vi "LoadDriveValues.vi"(8 "error in":errorcluster) -> (0 "error out":errorcluster)   [LabVIEW 2015]
uses:
  Drive/Implementation/Advanced Drive VIs/PID Type Def.ctl
  <vilib>/Rock Robotics/Network Tables/NT Read Numeric Array.vi
  Drive/Implementation/RobotDriveGlobal.vi
panel:
  out "Speed PID":T1
  out "Distance PID":T1
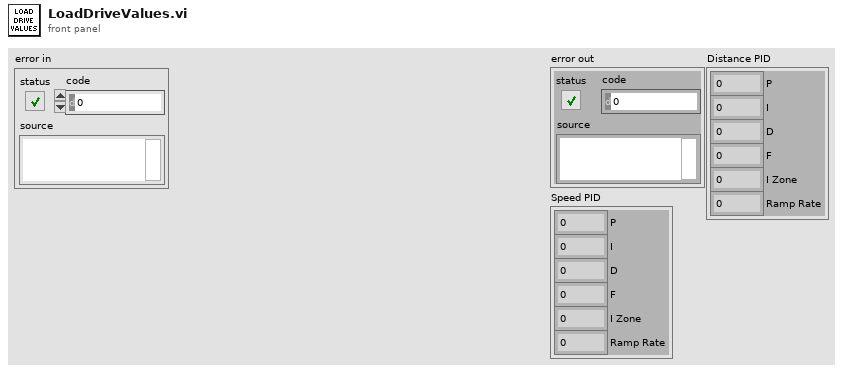
[diagram p1: front panel]
types:
  T1 = typedef "PID Type Def.ctl" = cluster{"P":dbl, "I":dbl, "D":dbl, "F":dbl, "I Zone":dbl, "Ramp Rate":dbl}
  T2 = typedef "RobotDrive Type Def.ctl" = cluster{"RobotDriveDevRef":cluster{"DevStatus":errorcluster, "Motors[]":T3[], "Square Inputs":bool, "Max Output":dbl}, "Control Mode":T9, "Motor Settings":T10, "Default Control Mode":T9, "Speed Mag":dbl}
  T3 = typedef "WPI_MotorControlDeviceRef.ctl" = cluster{"DeviceStatus":errorcluster, "Type":T4, "PWM":cluster{"PWM Channel":T5, "DeadBand":T6}, "CAN":cluster{"Device Number":u8, "Control Mode":T7, "Semaphore":T8, "Max Vout":dbl, "TalonSRX Control Mode":T9}, "Invert":bool}
  T4 = typedef "WPI_MotorControlType.ctl" = enum16{"PWM", "CAN", "CANTalonSRX"}
  T5 = typedef "FPGA_DIOPWMChannel.ctl" = enum8{"PWM 0", "PWM 1", "PWM 2", "PWM 3", "PWM 4", "PWM 5", "PWM 6", "PWM 7", "PWM 8", "PWM 9", "PWM MXP 0", "PWM MXP 1", "PWM MXP 2", "PWM MXP 3", "PWM MXP 4", "PWM MXP 5", "PWM MXP 6", "PWM MXP 7", "PWM MXP 8", "PWM MXP 9", "Invalid"}
  T6 = typedef "WPI_PWMDeadband.ctl" = cluster{"Name":string, "maxPositivePwm":i32, "minPositivePwm":i32, "centerPwm":i32, "maxNegativePwm":i32, "minNegativePwm":i32, "angularRange":u16}
  T7 = typedef "WPI_CANJaguar_ControlMode.ctl" = enum8{"Percent VBus", "Current", "Speed", "Position", "Voltage"}
  T8 = typedef "Semaphore RefNum" = refnum<k1>
  T9 = typedef "WPI_CANTalonSRX_APIControlMode.ctl" = enum8{"Percent VBus", "Speed", "Position", "Slave", "Unchanged / Invalid", "Voltage Compensation", "Current", "Motion Profile"}
  T10 = typedef "Drive Motor Settings.ctl" = cluster{"Wheel Radius":dbl, "Encoder Ticks Per Rev":dbl, "Gear Ratio":dbl, "ClimbRev":dbl}
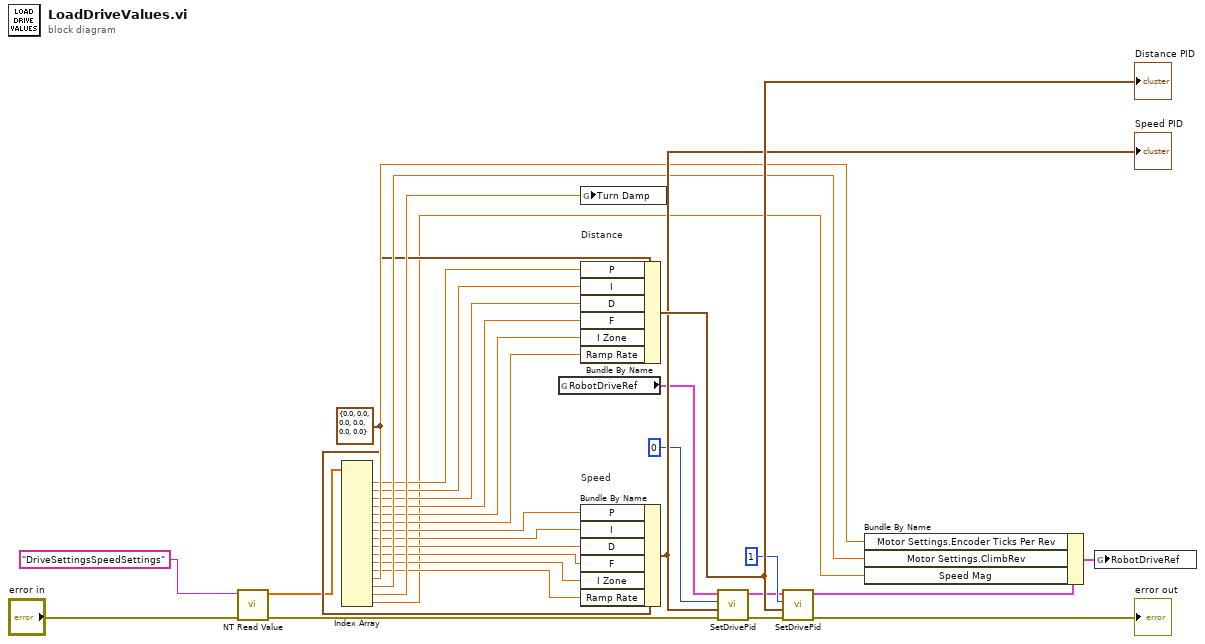
[diagram p0: block diagram]
diagram:
  w14 = T1 {"P"=0.0, "I"=0.0, "D"=0.0, "F"=0.0, "I Zone"=0.0, "Ramp Rate"=0.0} ("PID")
  n1 = call-poly <vilib>:"NT Read Value.vi"("error in"="error in", "Name"="DriveSettingsSpeedSettings") -> ("error out"=w3:errorcluster, "Numeric Array"=w7:dbl[])  [unwired: 8 in]
  n2 = Index Array(array=w7) -> (element #1=w8:dbl, element #2=w9:dbl, element #3=w10:dbl, element #4=w11:dbl, element #5=w12:dbl, element #6=w13:dbl, element #7=w15:dbl, element #8=w16:dbl, element #9=w17:dbl, element #10=w18:dbl, element #11=w19:dbl, element #12=w20:dbl, element #13=w28:dbl, element #14=w27:dbl, element #15=w31:dbl, element #16=w1:dbl)  [unwired: 16 in]
  n3 = global read "RobotDriveGlobal.vi" "RobotDriveRef"() -> (w21:T2)
  n4 = global write "RobotDriveGlobal.vi" "Turn Damp"(w31) -> ()
  n5 = Bundle By Name "Distance"(cluster=w14, "P"=w8, "I"=w9, "D"=w10, "F"=w11, "I Zone"=w12, "Ramp Rate"=w13) -> (w30:T1)
  "Distance PID" <- w30
  n6 = Bundle By Name "Speed"(cluster=w14, "P"=w15, "I"=w16, "D"=w17, "F"=w18, "I Zone"=w19, "Ramp Rate"=w20) -> (w29:T1)
  "Speed PID" <- w29
  n7 = call "SetDrivePid.vi"("error in (no error)"=w3, "PID"=w29, "Profile Slot"=u8 0, "RobotDriveRef In"=w21) -> ("error out"=w4:errorcluster, "RobotDriveRef Out"=w23:T2)  [unwired: 6 in]
  n8 = call "SetDrivePid.vi"("error in (no error)"=w4, "PID"=w30, "Profile Slot"=u8 1, "RobotDriveRef In"=w23) -> ("error out"=→"error out":errorcluster, "RobotDriveRef Out"=w25:T2)  [unwired: 6 in]
  n9 = Bundle By Name(cluster=w25, "Motor Settings.Encoder Ticks Per Rev"=w28, "Motor Settings.ClimbRev"=w27, "Speed Mag"=w1) -> (w26:T2)
  n10 = global write "RobotDriveGlobal.vi" "RobotDriveRef"(w26) -> ()
